vi "Debug_QueueTracker.vi"(7 "Mode":enum16{"Init", "Track", "DeInit"}(ring)=enum."Track", 8 "Error In":errorcluster, 10 "Message Cluster":T1, 11 "QueueIn":refnum<queue>) -> (0 "Error Out":errorcluster)   [LabVIEW 2017, in "Server.lvlib" / "Message Queue.lvlib"]
doc: "This VI is used to track all sent Queue-Messages in the Host Queued Message Handler. It receives the Message-Cluster adds some additional Data (Timestamp, Queue-Name, CallChain) and sends this information to a new Queue (\"TrackerQueue\"). This new Queue can now be read in the \"DebugCommunication.vi\" (in \"Tools\"-Folder) to display all messages an their data during execution.\nThis VI is for debugging purpouses only. You may consider to remove it from the code in the final version, but the code is very slim, so it shouldnt matter if you leave it."
uses:
  Message Queue.lvlib
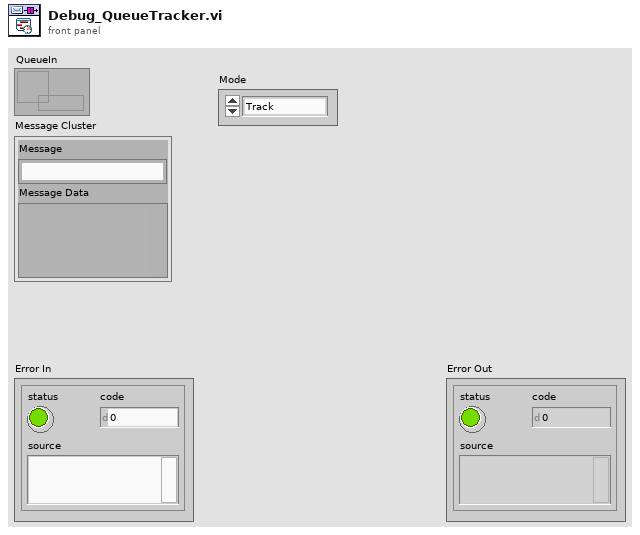
[diagram p1: front panel]
types:
  T1 = cluster{"Message":string, "Message Data":variant}
  T2 = cluster{"Time Stamp":timestamp, "Message Cluster":cluster{"Message":string, "Message Data":variant}, "CallChain":string[], "QueueName":string}
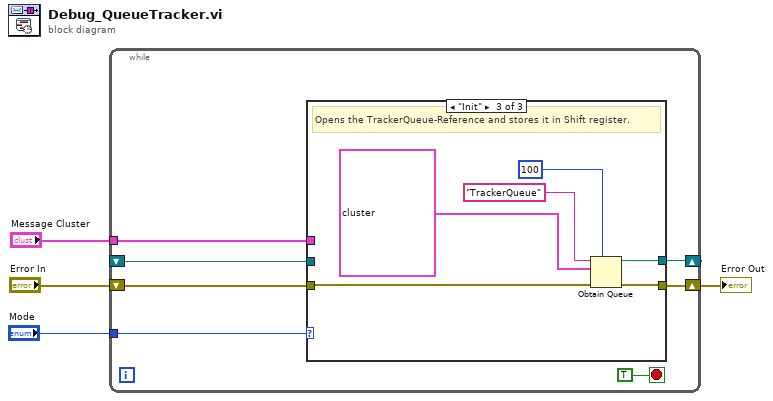
[diagram p0: block diagram]
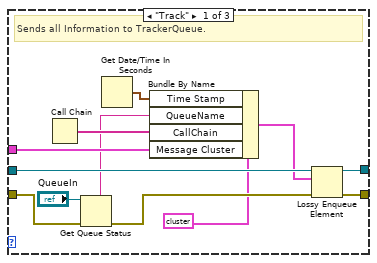
[diagram p2: hidden frame]
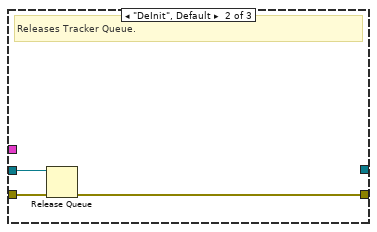
[diagram p3: hidden frame]
diagram:
  n1 = while {
    shift-right: [w10] -> _
    shift-left: _ -> [w9]
    shift-right: [w8] -> w3
    shift-left: "Error In" -> [w7]
    tunnel: "Message Cluster" -> [w6]
    tunnel: "Mode" -> [w5]
    stop <- TRUE stop-if-true
    n2 = case shown="\"Init\"" w5 {
      tunnel: [w21 _ w32] -> w10
      tunnel: w9 -> [w22 w24 _]
      tunnel: [w23 w25 w30] -> w8
      tunnel: w7 -> [w16 w26 w28]
      tunnel: w6 -> [w18 _ _]
      frame "Track" {
        # "Sends all Information to TrackerQueue."
        n3 = Call Chain() -> (call chain=w17:string[])
        n4 = Get Queue Status(queue="QueueIn", error in (no error)=w16) -> (queue name=w13:string, error out=w15:errorcluster)  [unwired: 1 in, 6 out]
        n5 = Get Date/Time In Seconds() -> (seconds since 1Jan1904=w20:timestamp)
        n6 = Bundle By Name(cluster=T2 {"Time Stamp"=timestamp(0 s since 1904-01-01), "Message Cluster"={"Message"="", "Message Data"=variant}, "CallChain"=[], "QueueName"=""} ("TrackerData"), "Time Stamp"=w20, "QueueName"=w13, "CallChain"=w17, "Message Cluster"=w18) -> (w19:T2)
        n7 = Lossy Enqueue Element(queue=w22, element=w19, error in (no error)=w15) -> (queue out=w21:refnum<queue>, error out=w23:errorcluster)  [unwired: 2 out]
      }
      frame "DeInit", Default {
        # "Releases Tracker Queue."
        n8 = Release Queue(queue=w24, error in (no error)=w26) -> (error out=w25:errorcluster)  [unwired: 1 in, 2 out]
      }
      frame "Init" {
        # "Opens the TrackerQueue-Reference and stores it in Shift register."
        n9 = Obtain Queue(max queue size (-1, unlimited)=100, name (unnamed)="TrackerQueue", element data type=T2 {"Time Stamp"=timestamp(0 s since 1904-01-01), "Message Cluster"={"Message"="", "Message Data"=variant}, "CallChain"=[], "QueueName"=""} ("TrackerData"), error in (no error)=w28) -> (queue out=w32:refnum<queue>, error out=w30:errorcluster)  [unwired: 1 in, 1 out]
      }
    }
  }
  "Error Out" <- w3
